vi "Average_Buffer_Scope.vi"(3 "N_Elements":i32, 4 "Index":i32, 5 "Buffersize":i32, 6 "Buffer in":cluster{"Diode":dbl, "Double Diode":dbl}[](array[cluster])) -> (1 "output devs":cluster{"Diode":dbl, "Double Diode":dbl}, 2 "output means":cluster{"Diode":dbl, "Double Diode":dbl})   [LabVIEW 2009]
uses:
  <vilib>/Analysis/NI_AALBase.lvlib
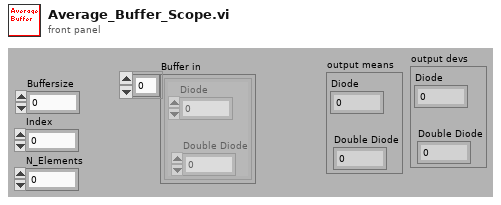
[diagram p1: front panel]
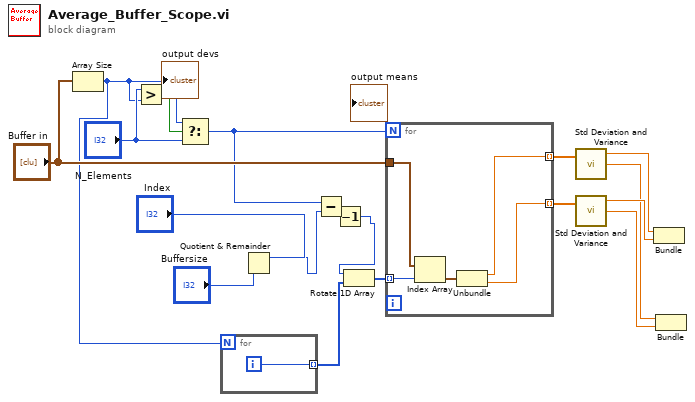
[diagram p0: block diagram]
diagram:
  n1 = Array Size(array="Buffer in") -> (size(s)=w5:i32)
  n2 = Greater?(x="N_Elements", y=w5) -> (0:w14:bool)
  n3 = Select(t=w5, s=w14, f="N_Elements") -> (s? t:f=w4:i32)
  n4 = for {
    N: w5 -> [_]
    tunnel: [w19] -> w10 mode=indexing
    i -> [w19]
  }
  n5 = Quotient & Remainder(x="Index", y="Buffersize") -> (x-y*floor(x/y)=w3:i32)  [unwired: 1 out]
  n6 = Subtract(x=w4, y=w3) -> (x-y=w2:i32)
  n7 = Decrement(x=w2) -> (x-1=w1:i32)
  n8 = Rotate 1D Array(1:w10, 2:w1) -> (0:w8:i32[])
  n9 = for {
    N: w4 -> [_]
    tunnel: [w21] -> w18 mode=indexing
    tunnel: [w20] -> w17 mode=indexing
    tunnel: "Buffer in" -> [w24]
    tunnel: w8 -> [w22] mode=indexing
    n10 = Index Array(array=w24, index=w22) -> (element=w23:cluster{"Diode":dbl, "Double Diode":dbl})
    n11 = Unbundle(w23) -> ("Diode"=w21:dbl, "Double Diode"=w20:dbl)
  }
  n12 = call <vilib>:"Std Deviation and Variance.vi"("X"=w18) -> ("mean"=w16:dbl, "standard deviation"=w7:dbl)  [unwired: 1 in, 1 out]
  n13 = call <vilib>:"Std Deviation and Variance.vi"("X"=w17) -> ("mean"=w15:dbl, "standard deviation"=w6:dbl)  [unwired: 1 in, 1 out]
  n14 = Bundle("mean"=w16, "mean"=w15) -> ()  [unwired: 1 in, 1 out]
  n15 = Bundle("standard deviation"=w7, "standard deviation"=w6) -> ()  [unwired: 1 in, 1 out]
